vi "WS1021 demo read error limits.vi"(8 "error in (no error)":errorcluster, 11 "file path (dialog if empty)":path) -> (0 "error out":errorcluster, 1 "Error limits":cluster{"Array":i32[], "Array":dbl[]}, 3 "new file path (Not A Path if cancelled)":path)   [LabVIEW 2020]
uses:
  <vilib>/Utility/file.llb/Read Delimited Spreadsheet (DBL).vi
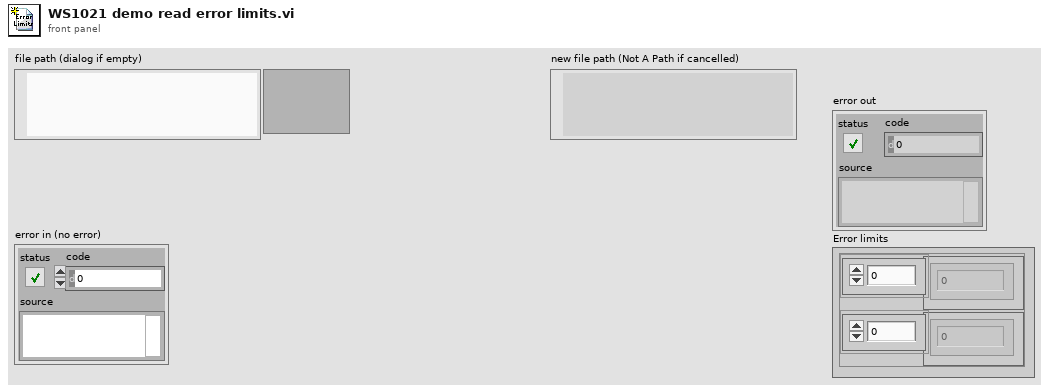
[diagram p1: front panel]
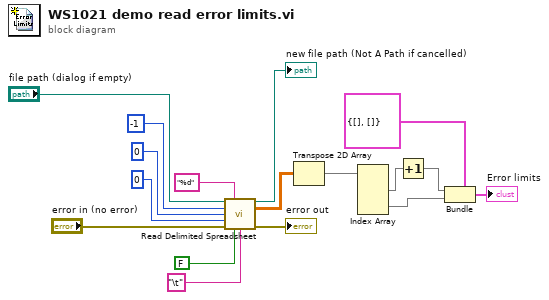
[diagram p0: block diagram]
diagram:
  n1 = call-poly <vilib>:"Read Delimited Spreadsheet.vi"("file path (dialog if empty)"="file path (dialog if empty)", "format (%.3f)"="%d", "number of rows (all:-1)"=-1, "start of read offset (chars.:0)"=0, "max characters/row  (no limit:0)"=0, "error in (no error)"="error in (no error)", "transpose? (F)"=FALSE, "delimiter (\\t)"="\t" ("delimiter (\\t)")) -> ("new file path (Not A Path if cancelled)"=→"new file path (Not A Path if cancelled)":path, "all rows"=w4:dbl[][], "error out"=→"error out":errorcluster)  [unwired: 2 in, 3 out]
  n2 = Transpose 2D Array(2D array=w4) -> (transposed array=w3:dbl[][])
  n3 = Index Array(array=w3) -> (element #1=w2:dbl[], element #2=w6:dbl[])  [unwired: 4 in]
  n4 = Increment(x=w2) -> (x+1=w1:dbl[])
  n5 = Bundle(cluster=cluster{i32[], dbl[]} {[], []}, w1, w6) -> (→"Error limits":cluster{i32[], dbl[]})
